vi "超过50个备份文件就删除旧的.vi"(8 "error in (no error)":errorcluster caption="error in", 11 "Folder Path":path caption="文件夹路径") -> (0 "error out":errorcluster)   [LabVIEW 2016, in "数据传输系统-03.lvlib" / "自动更新.lvlib"]
panel:
  out "deleted path":path
  out "Number of Files":i32 caption="文件数"
  out "All Files in Dir":path[](array[path]) caption="目录中的所有文件"
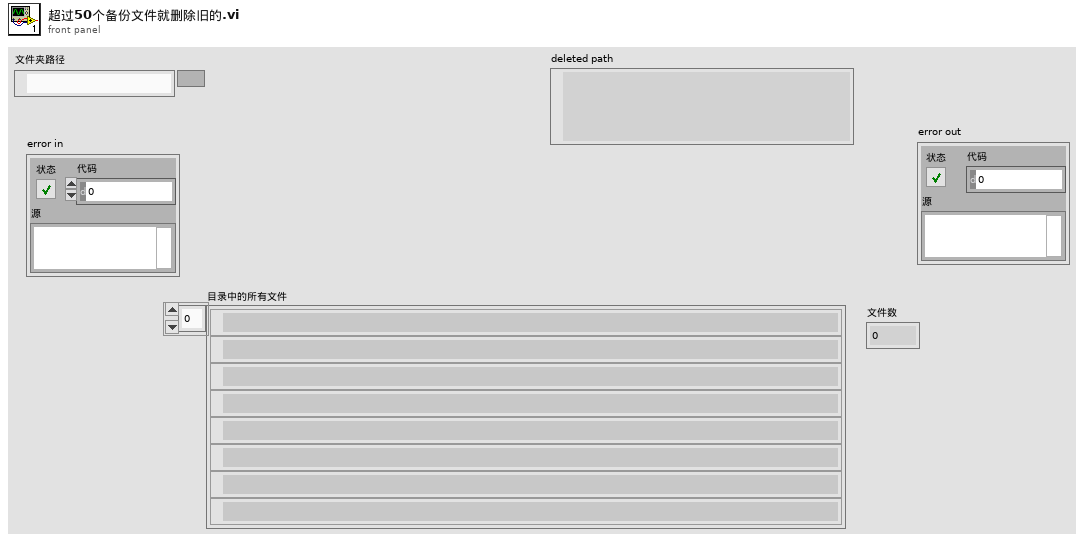
[diagram p1: front panel]
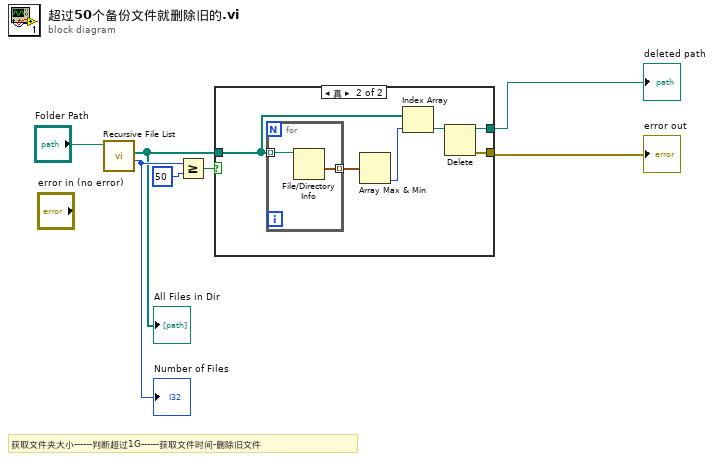
[diagram p0: block diagram]
diagram:
  # "获取文件夹大小------判断超过1G------获取文件时间-删除旧文件"
  n1 = call <vilib>:"Recursive File List.vi"("Folder Path"="Folder Path") -> ("Number of Files"=w7:i32, "All Files in Dir"=w3:path[])  [unwired: 6 in, 3 out]
  "Number of Files" <- w7
  "All Files in Dir" <- w3
  n2 = Greater Or Equal?(x=w7, y=50) -> (x >= y?=w2:bool)
  n3 = case shown="真" w2 {
    tunnel: w3 -> [_ w12]
    tunnel: [_ w9] -> w4
    tunnel: [_ w8] -> w5
    frame False {
    }
    frame True {
      n4 = for {
        tunnel: w12 -> [w15] mode=indexing
        tunnel: [w14] -> w13 mode=indexing
        n5 = File/Directory Info(path=w15) -> (last mod=w14:timestamp)  [unwired: 1 in, 6 out]
      }
      n6 = Array Max & Min(array=w13) -> (min index (indices)=w11:i32)  [unwired: 3 out]
      n7 = Index Array(array=w12, index=w11) -> (element=w10:path)
      n8 = Delete(path (use dialog)=w10) -> (deleted path=w9:path, error out=w8:errorcluster)  [unwired: 4 in, 1 out]
    }
  }
  "error out" <- w5
  "deleted path" <- w4
